vi "Configure Serial.vi"(8 "error in":errorcluster, 11 "MiniIO in":refnum<class "MiniIO.lvclass">) -> (0 "error out":errorcluster, 3 "MiniIO out":refnum<class "MiniIO.lvclass">)   [LabVIEW 2018, in "MiniIO.lvlib" / "MiniIO.lvclass"]
uses:
  MiniIO.lvclass
  MiniIO.lvclass/MiniIO.ctl
  PPLs/Configuration/Configuration.lvlibp/Configuration.lvclass
  PPLs/PLC/Parent/PLC.lvlibp/PLC.lvclass
  C:/AME Test Engineering/LabVIEW/PPLs/PLC/Parent/PLC.lvlibp/PLC.lvclass
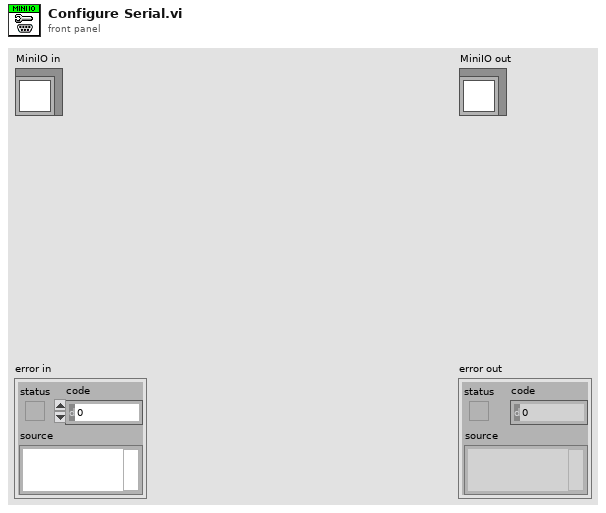
[diagram p1: front panel]
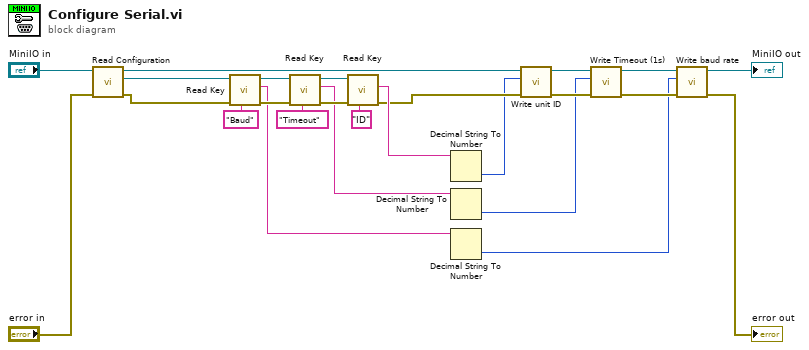
[diagram p0: block diagram]
diagram:
  n1 = call "Read Configuration.vi"("error in (no error)"="error in", "PLC in"="MiniIO in") -> ("error out"=w13:errorcluster, "Configuration"=w14:refnum<class "Configuration.lvclass">, "PLC out"=w11:refnum<class "MiniIO.lvclass">)  [unwired: 7 in]
  n2 = call "Read Key.vi"("Key:"="Baud", "error in"=w13, "Configuration in"=w14) -> ("error out"=w23:errorcluster, "Value"=w18:string, "Configuration out"=w22:refnum<class "Configuration.lvclass">)  [unwired: 6 in]
  n3 = call "Read Key.vi"("Key:"="Timeout", "error in"=w23, "Configuration in"=w22) -> ("error out"=w21:errorcluster, "Value"=w17:string, "Configuration out"=w20:refnum<class "Configuration.lvclass">)  [unwired: 6 in]
  n4 = call "Read Key.vi"("Key:"="ID", "error in"=w21, "Configuration in"=w20) -> ("error out"=w10:errorcluster, "Value"=w16:string)  [unwired: 6 in, 1 out]
  n5 = Decimal String To Number(string=w16) -> (number=w9:i32)  [unwired: 2 in, 1 out]
  n6 = Decimal String To Number(string=w17) -> (number=w2:i32)  [unwired: 2 in, 1 out]
  n7 = Decimal String To Number(string=w18) -> (number=w1:i32)  [unwired: 2 in, 1 out]
  n8 = call "Write unit ID.vi"("error in (no error)"=w10, "unit ID"=w9, "MiniIO in"=w11) -> ("error out"=w7:errorcluster, "MiniIO out"=w8:refnum<class "MiniIO.lvclass">)  [unwired: 7 in]
  n9 = call "Write Timeout (1s).vi"("error in (no error)"=w7, "Timeout (1s)"=w2, "MiniIO in"=w8) -> ("error out"=w5:errorcluster, "MiniIO out"=w6:refnum<class "MiniIO.lvclass">)  [unwired: 7 in]
  n10 = call "Write baud rate.vi"("error in (no error)"=w5, "baud rate"=w1, "MiniIO in"=w6) -> ("error out"=→"error out":errorcluster, "MiniIO out"=→"MiniIO out":refnum<class "MiniIO.lvclass">)  [unwired: 7 in]
